vi "Unflatten Compiled Data.vi"(8 "error in (no error)":errorcluster, 9 "Compiled.Settings":T6 {"Inline Execution Unit Compiled Information"."Outgoing Data References"."Data Reference" format="%.0x"; "Inline Execution Unit Compiled Information"."Incoming Data References" format="%.0x"}, 10 "RTStateVariables in":T1 {"Inline Execution Units"."Outgoing Data References"."Data Reference" format="%.0x"; "Inline Execution Units"."Incoming Data References" format="%.0x"}, 11 "Item Ref in":T9 format="%.0x") -> (0 "error out":errorcluster, 2 "RTStateVariables out":T1 {"Inline Execution Units"."Outgoing Data References"."Data Reference" format="%.0x"; "Inline Execution Units"."Incoming Data References" format="%.0x"}, 3 "Item Ref out":T9 format="%.0x")   [LabVIEW 2020, in "AIM MIL-STD-1553 Engine.lvlib" / "Custom Device.lvlib"]
doc: "Unflatten Execution Units and Shared Resources that were created on the host machine and passed to the engine as a flattened binary string and stores a copy of the unflattened data in RTStateVariables."
uses:
  Custom Device.lvlib
  <vilib>/NI VeriStand/Custom Device API/Custom Device Item Ref.ctl
  RTStateVariables.ctl
  <vilib>/NI/NIVS Inline Async API/_VS Inline Async API/VS Inline Async API/VS Inline Async API.lvclass
  Interfaces/Shared Resources/Shared Resources.lvclass
  Inline Execution Unit Runtime Information.ctl
  Interfaces/Execution Unit/Execution Unit.lvclass
  <vilib>/NI VeriStand/Custom Device API/Data Reference.ctl
  <vilib>/NI VeriStand/Custom Device API/Block Data Reference.ctl
  Asynchronous Execution Unit Runtime Information.ctl
  Compiled.Settings.ctl
  Inline Execution Unit Compiled Information.ctl
  Asynchronous Execution Unit Compiled Information.ctl
  <vilib>/NI VeriStand/Custom Device API/Custom Device API.lvlib
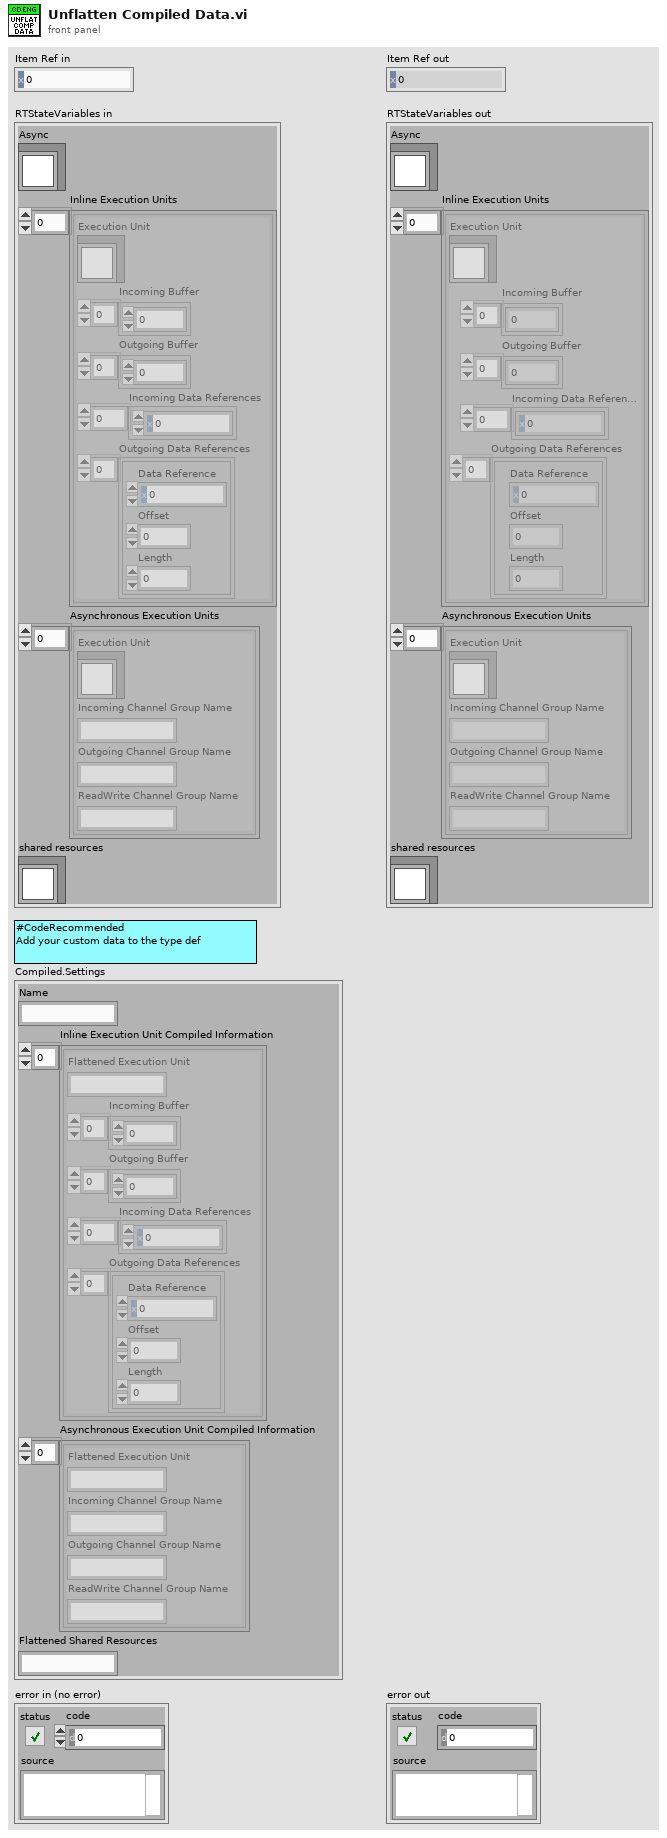
[diagram p1: front panel]
types:
  T1 = typedef "AIM MIL-STD-1553 Engine.lvlib/Custom Device.lvlib/RTStateVariables.ctl" = cluster{"Async":refnum<class "VS Inline Async API.lvclass">, "Inline Execution Units":T2[], "Asynchronous Execution Units":T5[], "shared resources":refnum<class "Shared Resources.lvclass">}
  T2 = typedef "AIM MIL-STD-1553 Engine.lvlib/Custom Device.lvlib/Inline Execution Unit Runtime Information.ctl" = cluster{"Execution Unit":refnum<class "Execution Unit.lvclass">, "Incoming Buffer":dbl[], "Outgoing Buffer":dbl[], "Incoming Data References":T3[], "Outgoing Data References":T4[]}
  T3 = typedef "Custom Device API.lvlib/Data Reference.ctl" = i32
  T4 = typedef "Custom Device API.lvlib/Block Data Reference.ctl" = cluster{"Data Reference":T3, "Offset":u64, "Length":u64}
  T5 = typedef "AIM MIL-STD-1553 Engine.lvlib/Custom Device.lvlib/Asynchronous Execution Unit Runtime Information.ctl" = cluster{"Execution Unit":refnum<class "Execution Unit.lvclass">, "Incoming Channel Group Name":string, "Outgoing Channel Group Name":string, "ReadWrite Channel Group Name":string}
  T6 = typedef "AIM MIL-STD-1553 Engine.lvlib/Custom Device.lvlib/Compiled.Settings.ctl" = cluster{"Name":string, "Inline Execution Unit Compiled Information":T7[], "Asynchronous Execution Unit Compiled Information":T8[], "Flattened Shared Resources":string}
  T7 = typedef "AIM MIL-STD-1553 Engine.lvlib/Custom Device.lvlib/Inline Execution Unit Compiled Information.ctl" = cluster{"Flattened Execution Unit":string, "Incoming Buffer":dbl[], "Outgoing Buffer":dbl[], "Incoming Data References":T3[], "Outgoing Data References":T4[]}
  T8 = typedef "AIM MIL-STD-1553 Engine.lvlib/Custom Device.lvlib/Asynchronous Execution Unit Compiled Information.ctl" = cluster{"Flattened Execution Unit":string, "Incoming Channel Group Name":string, "Outgoing Channel Group Name":string, "ReadWrite Channel Group Name":string}
  T9 = typedef "Custom Device API.lvlib/Custom Device Item Ref.ctl" = u64
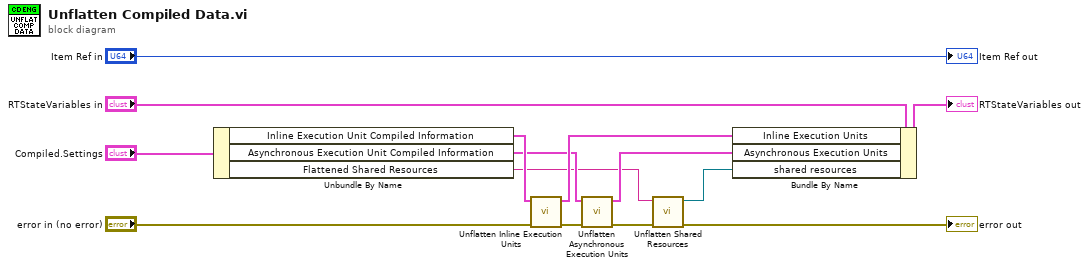
[diagram p0: block diagram]
diagram:
  n1 = Unbundle By Name("Compiled.Settings") -> ("Inline Execution Unit Compiled Information"=w9:T7[], "Asynchronous Execution Unit Compiled Information"=w8:T8[], "Flattened Shared Resources"=w3:string)
  n2 = call "Unflatten Inline Execution Units.vi"("error in (no error)"="error in (no error)", "Compiled Inline Execution Units"=w9) -> ("error out"=w6:errorcluster, "Inline Execution Units"=w10:T2[])  [unwired: 8 in]
  n3 = call "Unflatten Asynchronous Execution Units.vi"("error in (no error)"=w6, "Compiled Asynchronous Execution Units"=w8) -> ("error out"=w5:errorcluster, "Asynchronous Execution Units"=w7:T5[])  [unwired: 8 in]
  n4 = call "Unflatten Shared Resources.vi"("error in"=w5, "flattened shared resources"=w3) -> ("error out"=→"error out":errorcluster, "shared resources"=w2:refnum<class "Shared Resources.lvclass">)  [unwired: 8 in]
  n5 = Bundle By Name(cluster="RTStateVariables in", "Inline Execution Units"=w10, "Asynchronous Execution Units"=w7, "shared resources"=w2) -> (→"RTStateVariables out":T1)
  "Item Ref out" <- "Item Ref in"
